vi "testAssertionFailureMessage.vi"() -> ()   [LabVIEW 2019, in "AssertionTest.lvlib" / "AssertErrorCode.lvlib"]
uses:
  AssertErrorCode.lvlib
  <vilib>/Utility/error.llb/Error Cluster From Error Code.vi
  <vilib>/ErrorRing/Error Ring.xnode
  Assertion/Assertion.lvlib
panel:
  out "error out":errorcluster
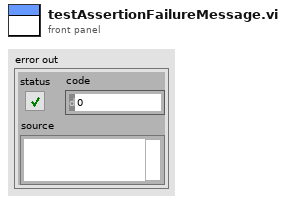
[diagram p1: front panel]
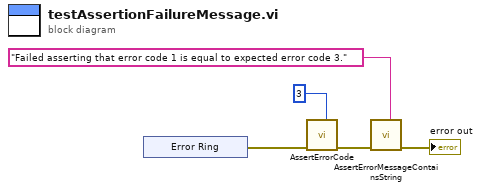
[diagram p0: block diagram]
diagram:
  n1 = xnode "Error Ring"() -> ("error out"=w5:errorcluster)
  n2 = call "AssertErrorCode.vi"("Expected"=3, "error in (no error)"=w5) -> ("error out"=w1:errorcluster)  [unwired: 9 in]
  n3 = call "AssertErrorMessageContainsString.vi"("Expected"="Failed asserting that error code 1 is equal to expected error code 3." ("Needle"), "error in (no error)"=w1) -> ("error out"=→"error out":errorcluster)  [unwired: 9 in]
